vi "Serial Output Test.vi"() -> ()   [LabVIEW 2011]
uses:
  <vilib>/Instr/_visa.llb/VISA Configure Serial Port (Instr).vi
panel:
  in  "VISA resource name":refnum<visa-resource-name>
  out "return count":u32
  in  "stop":bool
  out "unsigned byte array":u8[](array[numeric])
  out "read buffer":string
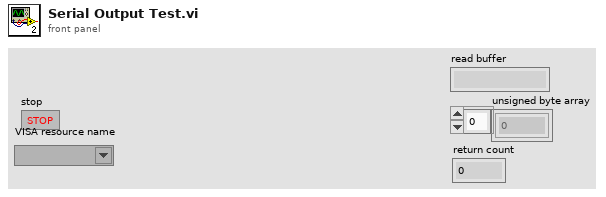
[diagram p1: front panel]
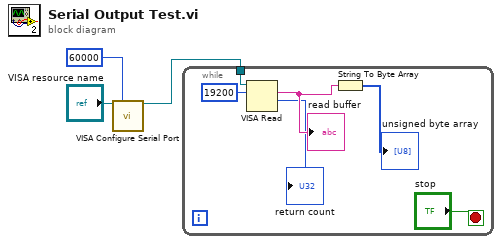
[diagram p0: block diagram]
diagram:
  n1 = call-poly "VISA Configure Serial Port"("VISA resource name"="VISA resource name", "timeout (10sec)"=u32 60000) -> ("VISA resource name out"=w1:refnum<visa-resource-name>)  [unwired: 12 in, 1 out]
  n2 = while {
    tunnel: w1 -> [w4]
    stop <- "stop" stop-if-true
    n3 = VISA Read(VISA resource name=w4, byte count=u32 19200) -> (read buffer=w8:string, return count=→"return count":u32)  [unwired: 1 in, 2 out]
    "read buffer" <- w8
    n4 = String To Byte Array(string=w8) -> (unsigned byte array=→"unsigned byte array":u8[])
  }
